vi "Wait Until Cancelled or Complete.vi"(6 "done channel":T1, 8 "error in (no error)":errorcluster, 9 "ms polling interval":i32=100, 11 "measure call context in":refnum<class "Measure Call Context.lvclass">) -> (0 "error out":errorcluster, 3 "measure call context out":refnum<class "Measure Call Context.lvclass">)   [LabVIEW 2023, in "FPT Pulse Measurement.lvclass"]
doc: "Monitor for cancellation and abort the measurement if a cancellation request is received before the measurement completes normally."
uses:
  FPT Pulse Measurement.lvclass
  <vilib>/Plug-In SDKs/Measurements/Measure Call Context/Measure Call Context.lvclass
  <extravilib>/ChannelInstances/Event Messenger-bool/))Channel.ctl
  <extravilib>/ChannelInstances/Event Messenger-bool/))Channel.vi
  <extravilib>/ChannelInstances/Event Messenger-bool.lvlib
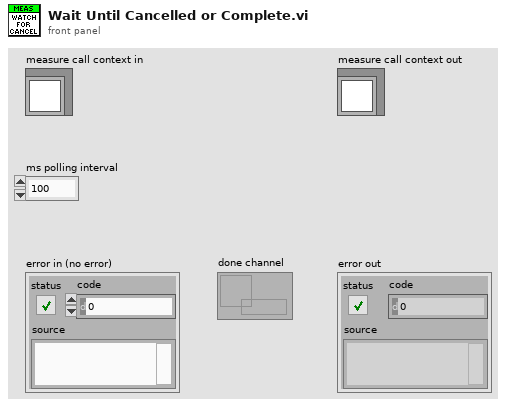
[diagram p1: front panel]
types:
  T1 = typedef "Event Messenger-bool.lvlib/))Channel.ctl" = refnum<queue>
  T2 = enum32{"Invalid", "Standard", "Closed", "Hidden", "Minimized", "Maximized"}
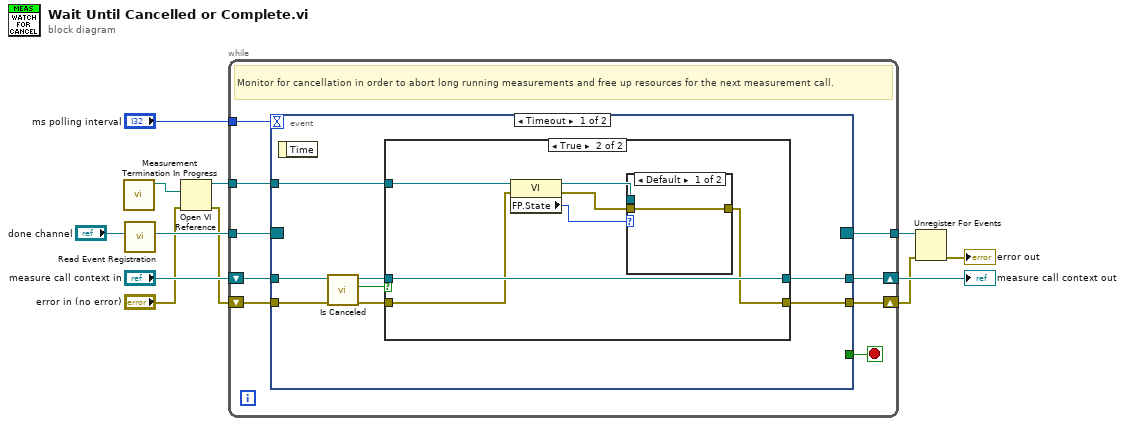
[diagram p0: block diagram]
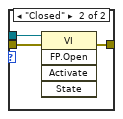
[diagram p3: hidden frame]
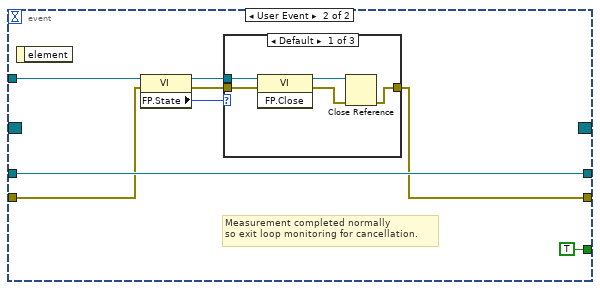
[diagram p4: hidden frame]
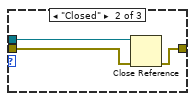
[diagram p5: hidden frame]
diagram:
  n1 = call "Measurement Termination In Progress.vi"() -> ("VI Path"=w4:path)  [unwired: 11 in]
  n2 = call <extravilib>:"Read Event Registration.vi"("channel"="done channel") -> ("event registration refnum"=w9:refnum<event-registration>)  [unwired: 10 in]
  n3 = Open VI Reference(vi path=w4, error in (no error)="error in (no error)") -> (vi reference=w3:refnum<vi>, error out=w1:errorcluster)  [unwired: 4 in]
  n4 = while {
    shift-right: [w20] -> w12
    shift-left: "measure call context in" -> [w21]
    shift-right: [w17] -> w6
    shift-left: w1 -> [w18]
    tunnel: w9 -> [w16]
    tunnel: "ms polling interval" -> [w15]
    tunnel: [w14] -> w7
    tunnel: w3 -> [w13]
    stop <- w19 stop-if-true
    # "Monitor for cancellation in order to abort long running measurements and free up resources for the next measurement call."
    n5 = event shown="[0] Timeout" {
      selector: w16 -> [_ _]
      dyn-events: [_ _] -> w14
      timeout: w15 -> [_ _]
      tunnel: w21 -> [w29 w49]
      tunnel: [w28 w49] -> w20
      tunnel: [_ TRUE ("is canceled?")] -> w19
      tunnel: w18 -> [w26 w44]
      tunnel: [w25 w46] -> w17
      tunnel: w13 -> [w22 w48]
      event Timeout {
        n6 = event-data() -> ()  [unwired: 1 in, 1 out]
        n7 = call <vilib>:"Is Canceled.vi"("error in"=w26, "measure call context in"=w29) -> ("error out"=w24:errorcluster, "is canceled?"=w27:bool, "measure call context out"=w23:refnum<class "Measure Call Context.lvclass">)  [unwired: 7 in]
        n8 = case shown="True" w27 {
          tunnel: w24 -> [w31 w32]
          tunnel: w23 -> [w30 w38]
          tunnel: [w31 w34] -> w25
          tunnel: [w30 w38] -> w28
          tunnel: w22 -> [_ w33]
          frame False {
          }
          frame True {
            n9 = property class="VI"(reference=w33, error in=w32) -> (reference out=w36:refnum<vi>, error out=w37:errorcluster, "FP.State"=w35:T2)
            n10 = case shown="Default" w35 {
              tunnel: w37 -> [w39 w42]
              tunnel: w36 -> [_ w41]
              tunnel: [w39 w40] -> w34
              frame Default {
              }
              frame "Closed" {
                n11 = invoke class="VI" method="FP.Open"(reference=w41, error in=w42) -> (error out=w40:errorcluster)  [unwired: 3 in, 4 out]
              }
            }
          }
        }
      }
      event User Event {
        # "Measurement completed normally\nso exit loop monitoring for cancellation."
        n12 = event-data() -> ()  [unwired: 1 in, 1 out]
        n13 = property class="VI"(reference=w48, error in=w44) -> (reference out=w47:refnum<vi>, error out=w45:errorcluster, "FP.State"=w43:T2)
        n14 = case shown="Default" w43 {
          tunnel: w45 -> [w55 w58 w59]
          tunnel: w47 -> [w54 w57 _]
          tunnel: [w51 w56 w59] -> w46
          frame Default {
            n15 = invoke class="VI" method="FP.Close"(reference=w54, error in=w55) -> (reference out=w52:refnum<vi>, error out=w53:errorcluster)  [unwired: 1 in, 1 out]
            n16 = Close Reference(reference=w52, error in (no error)=w53) -> (error out=w51:errorcluster)
          }
          frame "Closed" {
            n17 = Close Reference(reference=w57, error in (no error)=w58) -> (error out=w56:errorcluster)
          }
          frame "Invalid" {
          }
        }
      }
    }
  }
  "measure call context out" <- w12
  n18 = Unregister For Events(event registration refnum=w7, error in=w6) -> (error out=→"error out":errorcluster)
